vi "题目2.vi"() -> ()   [LabVIEW 2017]
panel:
  out "注册":bool
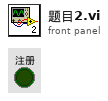
[diagram p1: front panel]
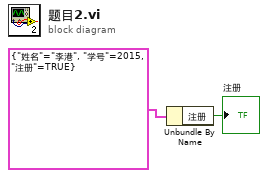
[diagram p0: block diagram]
diagram:
  n1 = Unbundle By Name(cluster{"姓名":string, "学号":i32, "注册":bool} {"姓名"="李港", "学号"=2015, "注册"=TRUE}) -> ("注册"=→"注册":bool)
